vi "lab2_3.vi"() -> ()   [LabVIEW 2026]
uses:
  <vilib>/express/express analysis/Spectral/Block/exnSpectralBlock spectral measurements RMS poly.vi
  <vilib>/express/express analysis/Spectral/Block/exnSpectralBlock spectral measurements RMS DDT.vi
  <vilib>/express/express analysis/Spectral/XNode/ExpressSpectralMeasurementsBlockNode.xnode
panel:
  out "Intensity Chart":dbl[][](graph)
  out "Waveform Graph 2":dynamicdata(graph)
  out "Waveform Graph":dynamicdata(graph)
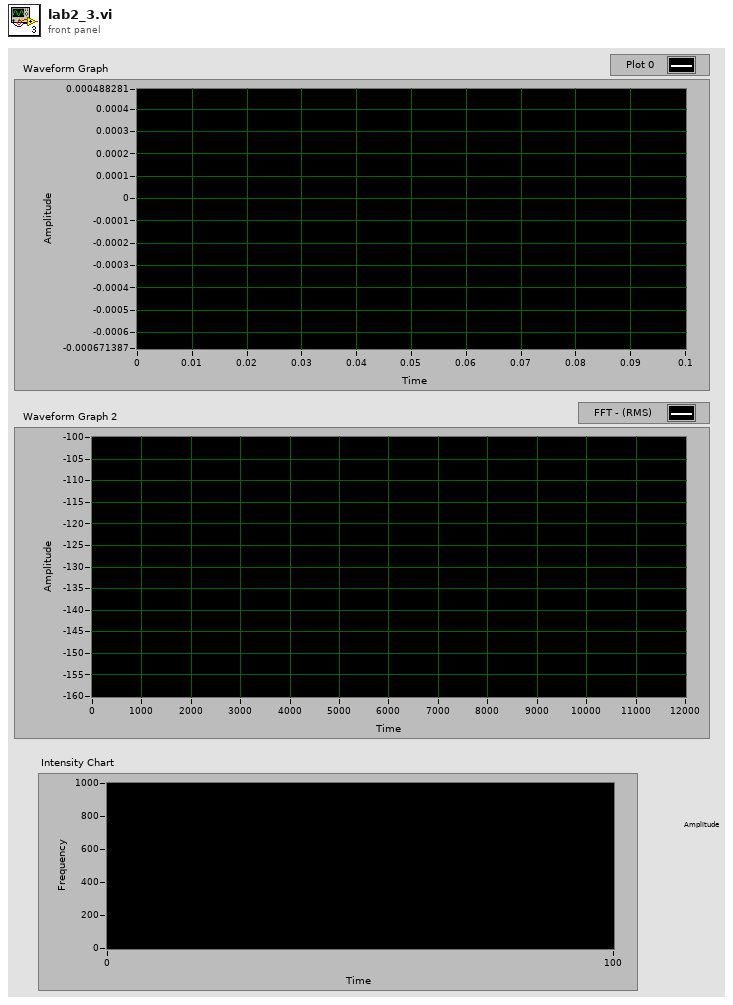
[diagram p1: front panel]
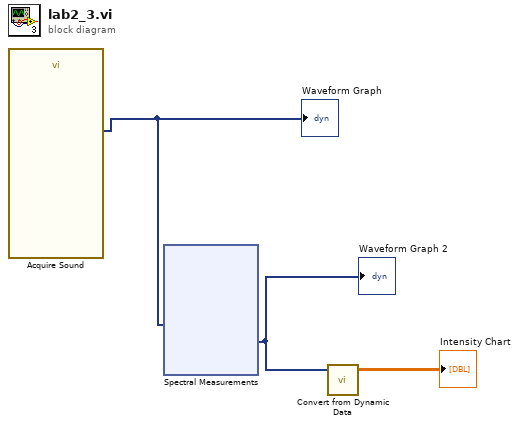
[diagram p0: block diagram]
diagram:
  n1 = call "Acquire Sound"() -> ("Data"=w3:dynamicdata)  [unwired: 18 in, 1 out]
  "Waveform Graph" <- w3
  n2 = xnode "Spectral Measurements"("Signals"=w3) -> ("FFT - (RMS)"=w2:dynamicdata)  [unwired: 1 in, 2 out]
  "Waveform Graph 2" <- w2
  n3 = call "Convert from Dynamic Data"("Dynamic Data Type"=w2) -> ("Array"=→"Intensity Chart":dbl[][])  [unwired: 3 in]
